vi "AlliGator Convert Phasor Value to Phasor Image Coordinates (N).vi"(8 "Phasor Plot Reference Points":T1, 10 "Phasor s":dbl[](array[numeric]), 11 "Phasor g":dbl[](array[numeric])) -> (2 "Phasor Plot y":i32[](array[numeric]), 3 "Phasor Plot x":i32[](array[numeric]))   [LabVIEW 2021, in "AlliGator Phasor Plot.lvlib"]
doc: "Converts array of phasor values to the corresponding array of Phasor Plot image coordinates."
uses:
  AlliGator Phasor Plot.lvlib
  AlliGator Phasor Plot Reference Points.ctl
  AlliGator Phasor Ratio.lvlib
panel:
  # "see the AlliGator License on the block diagram (Ctrl+E or Window:Show Block Diagram)"
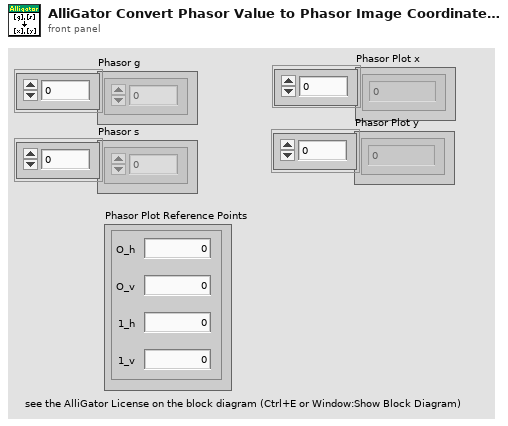
[diagram p1: front panel]
types:
  T1 = typedef "AlliGator Phasor Ratio.lvlib/AlliGator Phasor Plot Reference Points.ctl" = cluster{"O_h":dbl, "O_v":dbl, "1_h":dbl, "1_v":dbl}
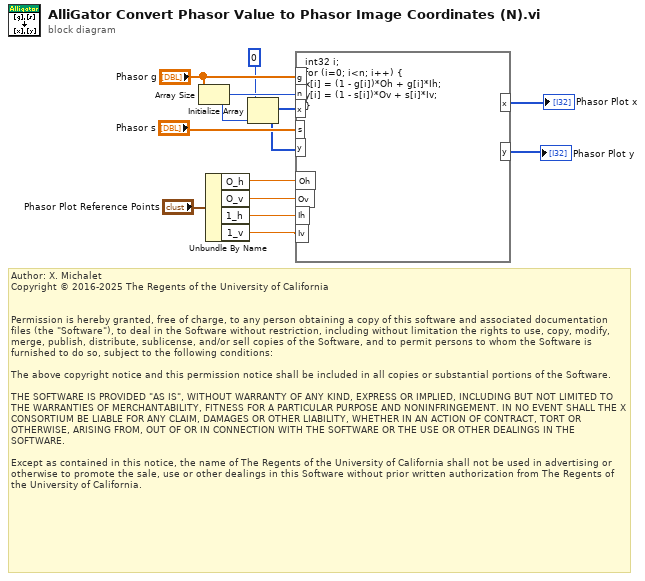
[diagram p0: block diagram]
diagram:
  # "Author: X. Michalet\nCopyright © 2016-2025 The Regents of the University of California\n \n\nPermission is hereby granted, free of charge, to any person obtaining a copy of this software and associated documentation files (the \"Software\"), to deal in the Software without restriction, including without limitation the rights to use, copy, modify, merge, publish, distribute, sublicense, and/or sell copies of the Software, and to permit persons to whom the Software is furnished to do so, subject to the following conditions:\n\nThe above copyright notice and this permission notice shall be included in all copies or substantial portions of the Software.\n\nTHE SOFTWARE IS PROVIDED \"AS IS\", WITHOUT WARRANTY OF ANY KIND, EXPRESS OR IMPLIED, INCLUDING BUT NOT LIMITED TO THE WARRANTIES OF MERCHANTABILITY, FITNESS FOR A PARTICULAR PURPOSE AND NONINFRINGEMENT. IN NO EVENT SHALL THE X CONSORTIUM BE LIABLE FOR ANY CLAIM, DAMAGES OR OTHER LIABILITY, WHETHER IN AN ACTION OF CONTRACT, TORT OR OTHERWISE, ARISING FROM, OUT OF OR IN CONNECTION WITH THE SOFTWARE OR THE USE OR OTHER DEALINGS IN THE SOFTWARE.\n\nExcept as contained in this notice, the name of The Regents of the University of California shall not be used in advertising or otherwise to promote the sale, use or other dealings in this Software without prior written authorization from The Regents of the University of California."
  n1 = Array Size(array="Phasor g") -> (size(s)=w3:i32)
  n2 = Unbundle By Name("Phasor Plot Reference Points") -> ("O_h"=w11:dbl, "O_v"=w10:dbl, "1_h"=w9:dbl, "1_v"=w8:dbl)
  n3 = Initialize Array(0 ("Phasor Plot x"), w3) -> (w1:i32[])
  n4 = formula code="int32 i;\nfor (i=0; i<n; i++) {\nx[i] = (1 - g[i])*Oh + g[i]*Ih;\ny[i] = (1 - s[i])*Ov + s[i]*Iv;\n}"("g"="Phasor g", "s"="Phasor s", "Oh"=w11, "Ov"=w10, "Ih"=w9, "Iv"=w8, "n"=w3, "x"=w1, "y"=w1) -> ("x"=→"Phasor Plot x":i32[], "y"=→"Phasor Plot y":i32[])
